vi "Tree Get Tokens.vi"(0 "ParseGDSII in":refnum<class "ParseGDSII.lvclass">) -> (1 "Record Payloads":string[](array[string]), 2 "Record Types":string[](array[string]), 3 "ParseGDSII out":refnum<class "ParseGDSII.lvclass">)   [LabVIEW 2019, in "ParseGDSII.lvclass"]
uses:
  ParseGDSII.lvclass
  ParseGDSII.lvclass/ParseGDSII.ctl
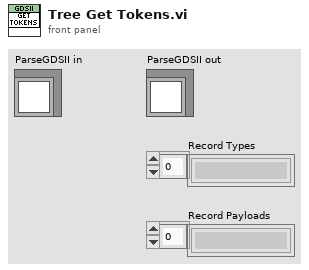
[diagram p1: front panel]
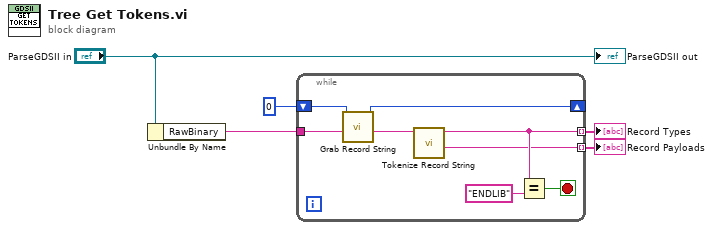
[diagram p0: block diagram]
diagram:
  n1 = Unbundle By Name("ParseGDSII in") -> ("RawBinary"=w3:string)
  n2 = while {
    tunnel: [w10] -> w2 mode=indexing
    tunnel: [w6] -> w1 mode=indexing
    shift-right: [w8] -> _
    shift-left: 0 ("New Offset") -> [w9]
    tunnel: w3 -> [w7]
    stop <- w11 stop-if-true
    n3 = call "Grab Record String.vi"("Raw Binary String"=w7, "Offset"=w9) -> ("Record String"=w12:string, "New Offset"=w8:i32)  [unwired: 8 in]
    n4 = call "Tokenize Record String.vi"("Record String"=w12) -> ("Payload Binary"=w6:string, "Record Type"=w10:string)  [unwired: 8 in, 1 out]
    n5 = Equal?(x=w10, y="ENDLIB") -> (x = y?=w11:bool)
  }
  "Record Types" <- w2
  "Record Payloads" <- w1
  "ParseGDSII out" <- "ParseGDSII in"
